vi "GetSpeedCmd.vi"(11 "Speed":dbl) -> (3 "Cmds":string[](array[string]))   [LabVIEW 2015]
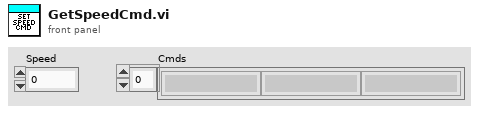
[diagram p1: front panel]
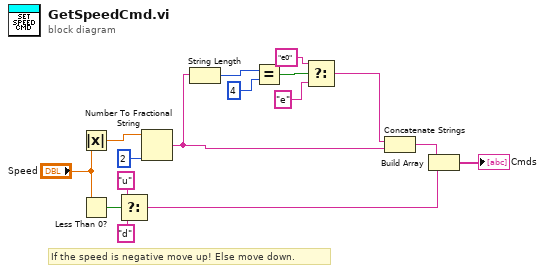
[diagram p0: block diagram]
diagram:
  # "If the speed is negative move up! Else move down."
  n1 = Absolute Value(x="Speed") -> (abs(x)=w8:dbl)
  n2 = Less Than 0?(x="Speed") -> (x < 0?=w10:bool)
  n3 = Select(t="u", s=w10, f="d") -> (s? t:f=w15:string)
  n4 = Number To Fractional String(number=w8, precision (6)=i16 2 ("width (-)")) -> (F-format string=w2:string)  [unwired: 2 in]
  n5 = String Length(string=w2) -> (length=w3:i32)
  n6 = Equal?(x=w3, y=4) -> (x = y?=w5:bool)
  n7 = Select(t="e0", s=w5, f="e") -> (s? t:f=w1:string)
  n8 = Concatenate Strings(w1, w2) -> (w14:string)
  n9 = Build Array(w14, w15) -> (→"Cmds":string[])
